vi "3D-ResetTotalNumber.vi"(10 "Inputs_BaseParam":string[](array[string]), 11 "名称或相对路径":string="UserDefine.ini") -> ()   [LabVIEW 2017]
uses:
  Global System.vi
  <vilib>/Utility/config.llb/NI_LVConfig.lvlib
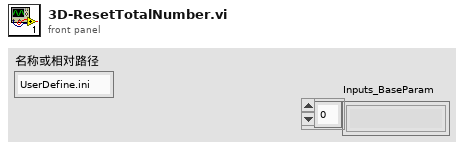
[diagram p1: front panel]
types:
  T1 = typedef "NI_LVConfig.lvlib/Config Data RefNum.ctl" = refnum<k1>
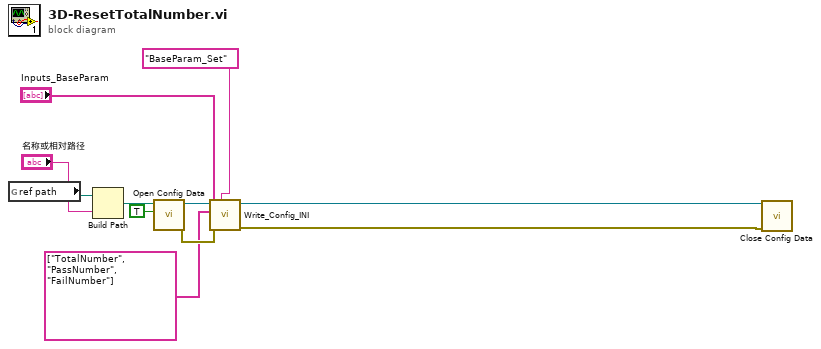
[diagram p0: block diagram]
diagram:
  n1 = global read "Global System.vi" "ref path"() -> (w6:path)
  n2 = Build Path(base path=w6, name or relative path="名称或相对路径") -> (appended path=w4:path)
  n3 = call <vilib>:"Open Config Data.vi"("create file if necessary (T)"=TRUE, "configuration file path"=w4) -> ("error out"=w10:errorcluster, "refnum"=w9:T1)  [unwired: 7 in, 1 out]
  n4 = call "Write_Config_INI.vi"("section"="BaseParam_Set", "error in (no error)"=w10, "Inputs"="Inputs_BaseParam", "Keys"=string[] ["TotalNumber", "PassNumber", "FailNumber"], "refnum"=w9) -> ("error out"=w1:errorcluster, "refnum 2"=w2:T1)  [unwired: 5 in]
  n5 = call <vilib>:"Close Config Data.vi"("error in (no error)"=w1, "refnum"=w2) -> ()  [unwired: 8 in, 2 out]
